vi "Flush Measurements.vi"(8 "error in (no error)":errorcluster, 11 "VISA in":refnum<visa-resource-name>) -> (0 "error out":errorcluster, 3 "VISA out":refnum<visa-resource-name>)   [LabVIEW 2013, in "Counter.lvlib" / "PICOTEST U62XXA series.lvlib"]
doc: "Dump eventual measured unread data from a buffer."
uses:
  PICOTEST U62XXA series.lvlib
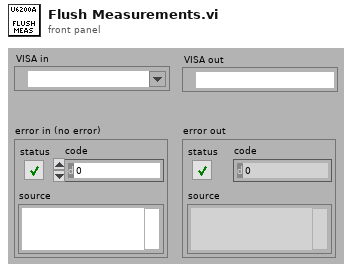
[diagram p1: front panel]
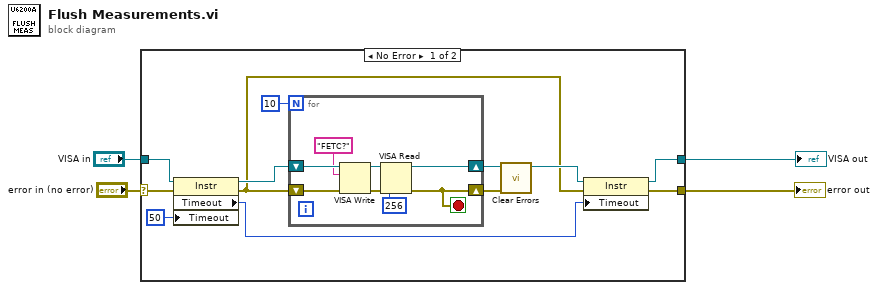
[diagram p0: block diagram]
diagram:
  n1 = case shown="No Error" "error in (no error)" {
    selector: "error in (no error)" -> [w5 w25]
    tunnel: "VISA in" -> [w15 w24]
    tunnel: [w10 w25] -> w3
    tunnel: [w9 w24] -> w2
    frame No Error {
      n2 = property class="Instr"(reference=w15, error in=w5, "Timeout"=u32 50 ("General Settings:Timeout Value")) -> (reference out=w13:refnum<visa-resource-name>, error out=w6:errorcluster, "Timeout"=w8:u32)
      n3 = for {
        N: 10 -> [_]
        shift-right: [w16] -> w12
        shift-left: w6 -> [w23]
        shift-right: [w17] -> w11
        shift-left: w13 -> [w22]
        stop <- w16 stop-if-true
        n4 = VISA Write(VISA resource name=w22, write buffer="FETC?", error in (no error)=w23) -> (VISA resource name out=w19:refnum<visa-resource-name>, error out=w20:errorcluster)  [unwired: 1 out]
        n5 = VISA Read(VISA resource name=w19, byte count=u32 256, error in (no error)=w20) -> (VISA resource name out=w17:refnum<visa-resource-name>, error out=w16:errorcluster)  [unwired: 2 out]
      }
      n6 = call <vilib>:"Clear Errors.vi"("error in (no error)"=w12) -> ()  [unwired: 6 in, 1 out]
      n7 = property class="Instr"(reference=w11, error in=w6, "Timeout"=w8) -> (reference out=w9:refnum<visa-resource-name>, error out=w10:errorcluster)
    }
    frame Error {
    }
  }
  "error out" <- w3
  "VISA out" <- w2
